vi "Network Operation.vi"(5 "AK?":bool, 7 "Operation":T1, 8 "error in (no error)":errorcluster, 10 "Message":string, 11 "Listener In.lvclass":refnum<class "Listener.lvclass">) -> (0 "error out":errorcluster, 3 "Listener Out.lvclass":refnum<class "Listener.lvclass">)   [LabVIEW 2019, in "Listener.lvclass"]
uses:
  Listener.lvclass
  ListenerClassControls/Operation Ctl.ctl
  <vilib>/Utility/error.llb/Error Cluster From Error Code.vi
  Protocols.lvlib
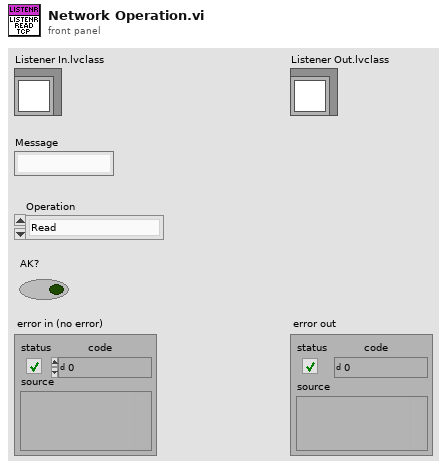
[diagram p1: front panel]
types:
  T1 = typedef "Operation Ctl.ctl" = enum16{"Read", "Write"}
  T2 = enum16{"Standard", "Buffered", "CRLF", "Immediate"}
  T3 = typedef "Listener.lvclass/Protocol Ctl.ctl" = enum16{"RS-XXX", "VISA", "TCPIP", "UDP", "GPIB ConvBox"}
  T4 = typedef "Listener.lvclass/UDP Data Structure.ctl" = cluster{"UDP connection ID":refnum<k16>, "Local Address":string, "Local Port":u16, "Target IP Address":string, "Target Port":u16, "Data":string}
  T5 = typedef "Listener.lvclass/TCP IP Data Structure.ctl" = cluster{"TCP|IP connection ID":refnum<k5>, "IP Address":string, "Port":u16, "Data":string}
  T6 = typedef "Listener.lvclass/AK TCP IP Data Structure.ctl" = cluster{"TCP|IP connection ID":refnum<k5>, "IP Address":string, "Port":u16, "Data":string, "Current Command Code":string}
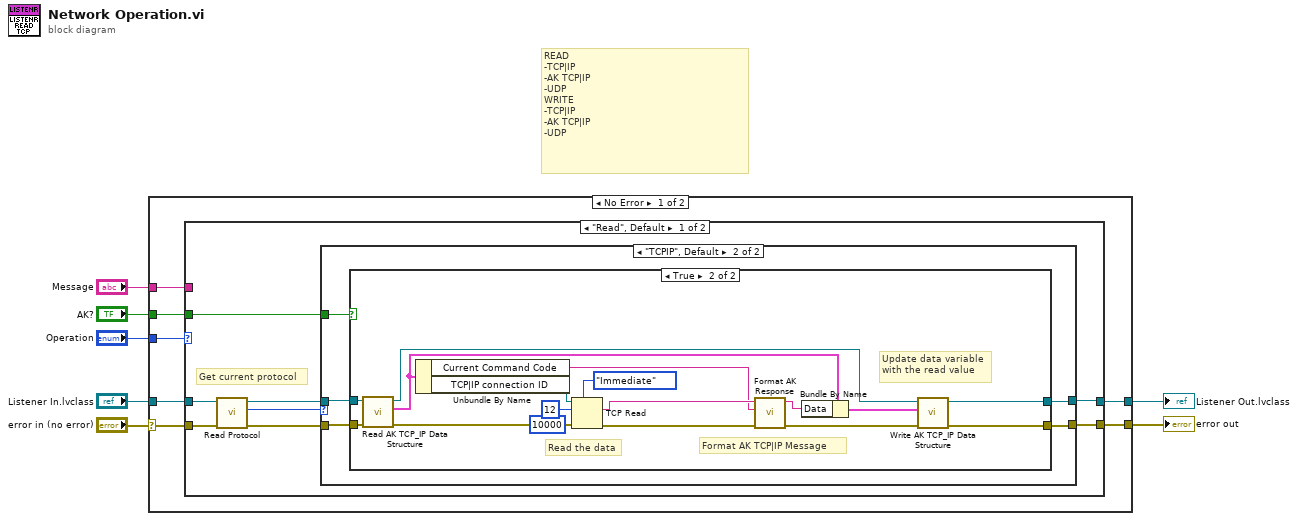
[diagram p0: block diagram]
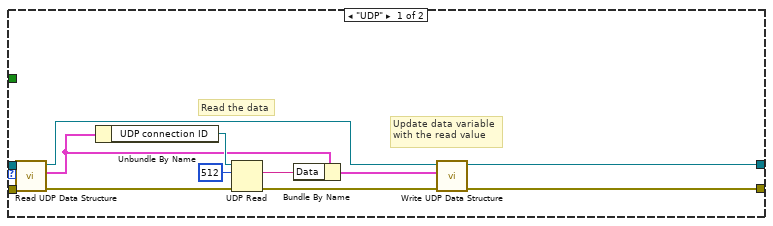
[diagram p2: hidden frame]
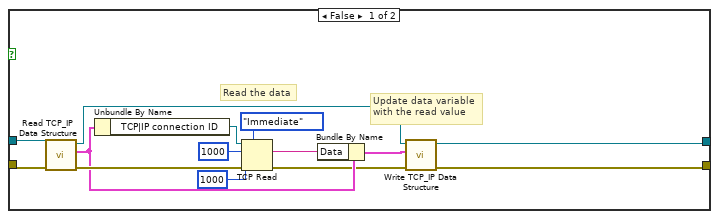
[diagram p3: hidden frame]
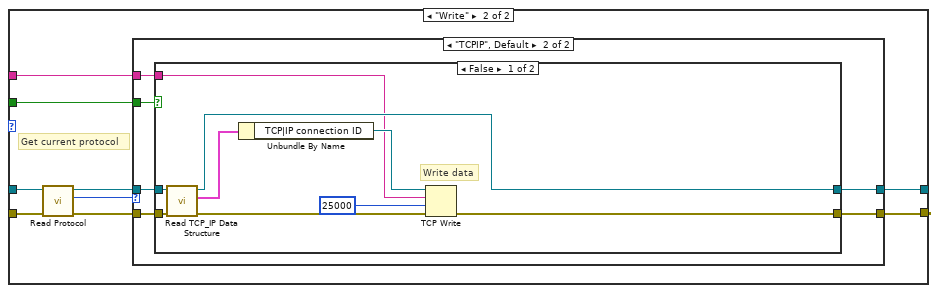
[diagram p4: hidden frame]
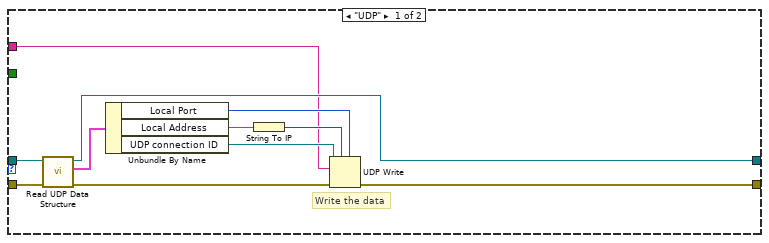
[diagram p5: hidden frame]
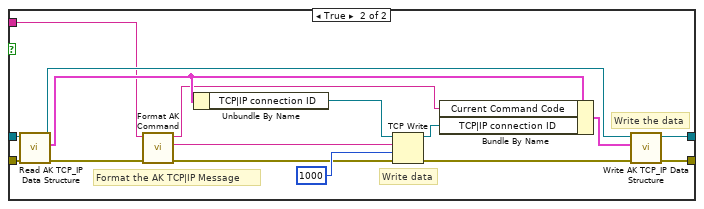
[diagram p6: hidden frame]
diagram:
  # "READ\n-TCP|IP\n-AK TCP|IP\n-UDP\nWRITE\n-TCP|IP\n-AK TCP|IP\n-UDP"
  n1 = case shown="No Error" "error in (no error)" {
    selector: "error in (no error)" -> [w11 w122]
    tunnel: "Listener In.lvclass" -> [w14 w123]
    tunnel: [w13 w122] -> w6
    tunnel: [w12 w123] -> w5
    tunnel: "Operation" -> [w10 _]
    tunnel: "AK?" -> [w9 _]
    tunnel: "Message" -> [w8 _]
    frame No Error {
      n2 = case shown="\"Read\", Default" w10 {
        tunnel: w11 -> [w22 w77]
        tunnel: w14 -> [w21 w74]
        tunnel: [w18 w78] -> w13
        tunnel: [w17 w79] -> w12
        tunnel: w9 -> [w15 w72]
        tunnel: w8 -> [_ w71]
        frame "Read", Default {
          # "Get current protocol"
          n3 = call-dynamic "Read Protocol.vi"("error in (no error)"=w22, "Listener in"=w21) -> ("error out"=w20:errorcluster, "Protocol"=w16:T3, "Listener out"=w19:refnum<class "Listener.lvclass">)  [unwired: 7 in]
          n4 = case shown="\"TCPIP\", Default" w16 {
            tunnel: w20 -> [w34 w39]
            tunnel: w19 -> [w33 w38]
            tunnel: [w31 w36] -> w17
            tunnel: [w32 w37] -> w18
            tunnel: w15 -> [_ w35]
            frame "UDP" {
              # "Read the data"
              # "Update data variable\nwith the read value"
              n5 = call-dynamic "Read UDP Data Structure.vi"("error in (no error)"=w34, "Listener in"=w33) -> ("error out"=w30:errorcluster, "UDP Data Structure"=w27:T4, "Listener out"=w24:refnum<class "Listener.lvclass">)  [unwired: 7 in]
              n6 = Unbundle By Name(w27) -> ("UDP connection ID"=w28:refnum<k16>)
              n7 = UDP Read(connection ID=w28, max size (548)=512, 8:w30) -> (data out=w26:string, error out=w25:errorcluster)  [unwired: 1 in, 3 out]
              n8 = Bundle By Name(cluster=w27, "Data"=w26) -> (w23:T4)
              n9 = call-dynamic "Write UDP Data Structure.vi"("error in (no error)"=w25, "UDP Data Structure"=w23, "Listener in"=w24) -> ("error out"=w32:errorcluster, "Listener out"=w31:refnum<class "Listener.lvclass">)  [unwired: 7 in]
            }
            frame "TCPIP", Default {
              n10 = case shown="True" w35 {
                tunnel: w39 -> [w44 w69]
                tunnel: w38 -> [w45 w68]
                tunnel: [w42 w56] -> w37
                tunnel: [w43 w55] -> w36
                frame False {
                  # "Update data variable\nwith the read value"
                  # "Read the data"
                  n11 = call-dynamic "Read TCP_IP Data Structure.vi"("error in (no error)"=w44, "Listener in"=w45) -> ("error out"=w52:errorcluster, "TCP|IP Data Structure"=w51:T5, "Listener out"=w47:refnum<class "Listener.lvclass">)  [unwired: 7 in]
                  n12 = Unbundle By Name(w51) -> ("TCP|IP connection ID"=w46:refnum<k5>)
                  n13 = TCP Read(connection ID=w46, bytes to read=1000, error in (no error)=w52, 7:T2."Immediate" ("mode (standard)"), 9:1000 ("timeout ms (25000)")) -> (data out=w50:string, error out=w48:errorcluster)  [unwired: 1 out]
                  n14 = Bundle By Name(cluster=w51, "Data"=w50) -> (w49:T5)
                  n15 = call-dynamic "Write TCP_IP Data Structure.vi"("error in (no error)"=w48, "TCP|IP Data Structure"=w49, "Listener in"=w47) -> ("error out"=w42:errorcluster, "Listener out"=w43:refnum<class "Listener.lvclass">)  [unwired: 7 in]
                }
                frame True {
                  # "Format AK TCP|IP Message"
                  # "Update data variable\nwith the read value"
                  # "Read the data"
                  n16 = call-dynamic "Read AK TCP_IP Data Structure.vi"("error in (no error)"=w69, "Listener in"=w68) -> ("error out"=w66:errorcluster, "TCP|IP Data Structure"=w63:T6, "Listener out"=w59:refnum<class "Listener.lvclass">)  [unwired: 7 in]
                  n17 = Unbundle By Name(w63) -> ("Current Command Code"=w54:string, "TCP|IP connection ID"=w67:refnum<k5>)
                  n18 = TCP Read(connection ID=w67, bytes to read=12, error in (no error)=w66, 7:T2."Immediate" ("mode (standard)"), 9:10000 ("timeout ms (25000)")) -> (data out=w64:string, error out=w65:errorcluster)  [unwired: 1 out]
                  n19 = call "Format AK Response.vi"("error in (no error)"=w65, "Current Command Code"=w54, "Response"=w64) -> ("error out"=w61:errorcluster, "Data"=w62:string)  [unwired: 7 in]
                  n20 = Bundle By Name(cluster=w63, "Data"=w62) -> (w60:T6)
                  n21 = call-dynamic "Write AK TCP_IP Data Structure.vi"("error in (no error)"=w61, "TCP|IP Data Structure"=w60, "Listener in"=w59) -> ("error out"=w56:errorcluster, "Listener out"=w55:refnum<class "Listener.lvclass">)  [unwired: 7 in]
                }
              }
            }
          }
        }
        frame "Write" {
          # "Get current protocol"
          n22 = call-dynamic "Read Protocol.vi"("error in (no error)"=w77, "Listener in"=w74) -> ("error out"=w76:errorcluster, "Protocol"=w73:T3, "Listener out"=w75:refnum<class "Listener.lvclass">)  [unwired: 7 in]
          n23 = case shown="\"TCPIP\", Default" w73 {
            tunnel: [w87 w96] -> w79
            tunnel: [w88 w95] -> w78
            tunnel: w75 -> [w89 w93]
            tunnel: w76 -> [w90 w94]
            tunnel: w72 -> [_ w92]
            tunnel: w71 -> [w80 w91]
            frame "UDP" {
              # "Write the data"
              n24 = call-dynamic "Read UDP Data Structure.vi"("error in (no error)"=w90, "Listener in"=w89) -> ("error out"=w84:errorcluster, "UDP Data Structure"=w86:T4, "Listener out"=w87:refnum<class "Listener.lvclass">)  [unwired: 7 in]
              n25 = Unbundle By Name(w86) -> ("Local Port"=w83:u16, "Local Address"=w82:string, "UDP connection ID"=w85:refnum<k16>)
              n26 = String To IP(1:w82) -> (0:w81:u32)
              n27 = UDP Write(address=w81, port or service name=w83, connection ID=w85, data in=w80, 8:w84) -> (error out=w88:errorcluster)  [unwired: 1 in, 1 out]
            }
            frame "TCPIP", Default {
              n28 = case shown="False" w92 {
                tunnel: [w105 w111] -> w96
                tunnel: [w104 w113] -> w95
                tunnel: w94 -> [w103 w118]
                tunnel: w93 -> [w102 w117]
                tunnel: w91 -> [w97 w106]
                frame False {
                  # "Write data"
                  n29 = call-dynamic "Read TCP_IP Data Structure.vi"("error in (no error)"=w103, "Listener in"=w102) -> ("error out"=w98:errorcluster, "TCP|IP Data Structure"=w100:T5, "Listener out"=w105:refnum<class "Listener.lvclass">)  [unwired: 7 in]
                  n30 = Unbundle By Name(w100) -> ("TCP|IP connection ID"=w101:refnum<k5>)
                  n31 = TCP Write(connection ID=w101, data in=w97, error in (no error)=w98, 9:25000 ("timeout ms (25000)")) -> (error out=w104:errorcluster)  [unwired: 2 out]
                }
                frame True {
                  # "Format the AK TCP|IP Message"
                  # "Write the data"
                  # "Write data"
                  n32 = call-dynamic "Read AK TCP_IP Data Structure.vi"("error in (no error)"=w118, "Listener in"=w117) -> ("error out"=w116:errorcluster, "TCP|IP Data Structure"=w112:T6, "Listener out"=w115:refnum<class "Listener.lvclass">)  [unwired: 7 in]
                  n33 = call "Format AK Command.vi"("error in (no error)"=w116, "String in"=w106) -> ("error out"=w119:errorcluster, "Command"=w110:string, "Command Code"=w109:string)  [unwired: 7 in]
                  n34 = Unbundle By Name(w112) -> ("TCP|IP connection ID"=w121:refnum<k5>)
                  n35 = TCP Write(connection ID=w121, data in=w110, error in (no error)=w119, 9:1000 ("timeout ms (25000)")) -> (connection ID out=w108:refnum<k5>, error out=w114:errorcluster)  [unwired: 1 out]
                  n36 = Bundle By Name(cluster=w112, "Current Command Code"=w109, "TCP|IP connection ID"=w108) -> (w107:T6)
                  n37 = call-dynamic "Write AK TCP_IP Data Structure.vi"("error in (no error)"=w114, "TCP|IP Data Structure"=w107, "Listener in"=w115) -> ("error out"=w113:errorcluster, "Listener out"=w111:refnum<class "Listener.lvclass">)  [unwired: 7 in]
                }
              }
            }
          }
        }
      }
    }
    frame Error {
    }
  }
  "Listener Out.lvclass" <- w5
  "error out" <- w6
